vi "Configure Bitfile.vi"(0 "USRP RIO device":T1, 5 "which bitfile":string(combo)="Time", 11 "error in":errorcluster) -> (4 "USRP RIO device":T1, 6 "bitfile":path, 15 "error out":errorcluster)   [LabVIEW 2021]
uses:
  <vilib>/userdefined/Silver/nirio_resource_slv.ctl
  <vilib>/Utility/error.llb/Error Cluster From Error Code.vi
  <vilib>/regexp/Match Regular Expression.xnode
  <vilib>/ErrorRing/Error Ring.xnode
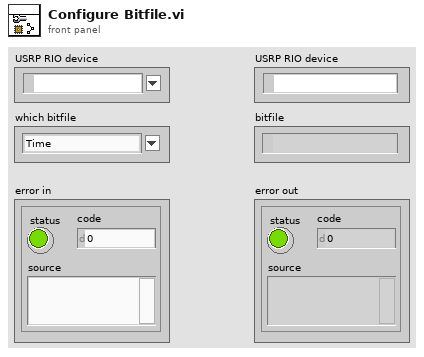
[diagram p1: front panel]
types:
  T1 = typedef "nirio_resource_slv.ctl" = tag
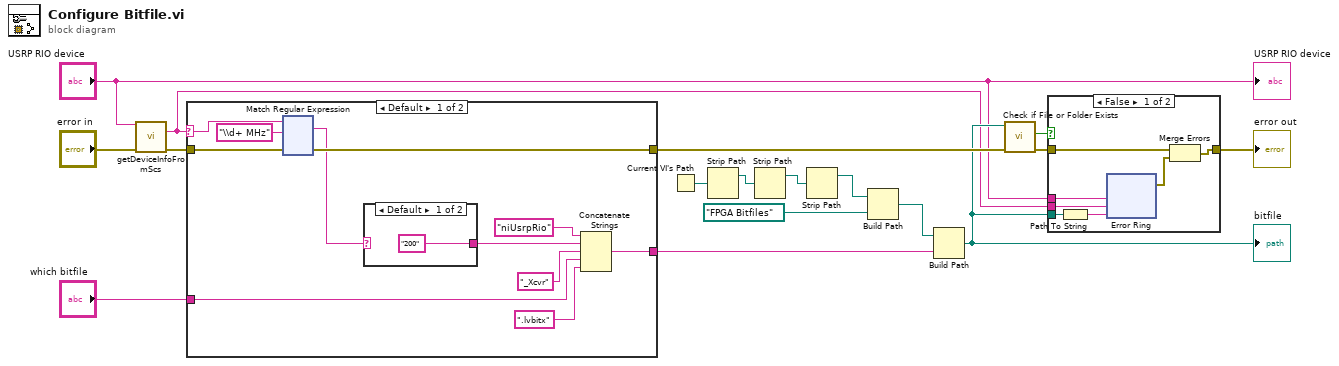
[diagram p0: block diagram]
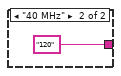
[diagram p3: hidden frame]
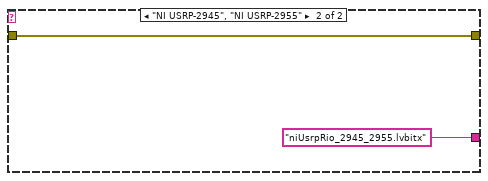
[diagram p4: hidden frame]
diagram:
  n1 = call <vilib>:"getDeviceInfoFromScs.vi"("rio device"="USRP RIO device", "error in"="error in") -> ("product name"=w5:string, "error out"=w9:errorcluster)  [unwired: 9 in, 3 out]
  n2 = case shown="Default" w5 {
    selector: w5 -> [w18 _]
    tunnel: "which bitfile" -> [w25 _]
    tunnel: w9 -> [w23 w148]
    tunnel: [w22 w148] -> w7
    tunnel: [w19 "niUsrpRio_2945_2955.lvbitx" ("f")] -> w8
    frame Default {
      n3 = xnode "Match Regular Expression"("input string"=w18, "regular expression"="\\d+ MHz", "error in"=w23) -> ("whole match"=w21:string, "error out"=w22:errorcluster)  [unwired: 3 in, 3 out]
      n4 = case shown="Default" w21 {
        tunnel: ["200" ("format string") "120" ("format string")] -> w20
        frame Default {
        }
        frame "40 MHz" {
        }
      }
      n5 = Concatenate Strings("niUsrpRio" ("format string"), w20, "_Xcvr" ("format string"), w25, ".lvbitx" ("format string")) -> (w19:string)
    }
    frame "NI USRP-2945", "NI USRP-2955" {
    }
  }
  n6 = Current VI's Path() -> (path=w17:path)
  n7 = Strip Path(path=w17) -> (stripped path=w14:path)  [unwired: 1 out]
  n8 = Strip Path(path=w14) -> (stripped path=w13:path)  [unwired: 1 out]
  n9 = Strip Path(path=w13) -> (stripped path=w12:path)  [unwired: 1 out]
  n10 = Build Path(base path=w12, name or relative path=path "FPGA Bitfiles") -> (appended path=w15:path)
  n11 = Build Path(base path=w15, name or relative path=w8) -> (appended path=w6:path)
  "bitfile" <- w6
  n12 = call <vilib>:"Check if File or Folder Exists.vi"("error in (no error)"=w7, "path"=w6) -> ("error out"=w2:errorcluster, "file or folder exists?"=w1:bool)  [unwired: 7 in, 1 out]
  n13 = case shown="False" w1 {
    tunnel: w6 -> [w156 _]
    tunnel: w5 -> [w154 _]
    tunnel: "USRP RIO device" -> [w153 _]
    tunnel: [w151 w166] -> w3
    tunnel: w2 -> [w152 w166]
    frame False {
      n14 = Path To String(path=w156) -> (string=w155:string)
      n15 = xnode "Error Ring"("parameter 0"=w153, "parameter 1"=w154, "parameter 2"=w155) -> ("error out"=w150:errorcluster)
      n16 = Merge Errors(w152, w150) -> (w151:errorcluster)
    }
    frame True {
    }
  }
  "error out" <- w3
  "USRP RIO device" <- "USRP RIO device"
